vi "CalculateInputString_v2.vi"(1 "InputString":string="1 + 2 * 4") -> (0 "result":dbl format="%.2f")   [LabVIEW 2018]
uses:
  <vilib>/gmath/NI_Gmath.lvlib
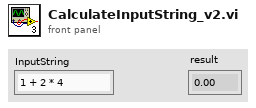
[diagram p1: front panel]
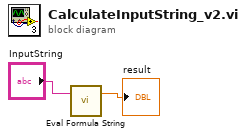
[diagram p0: block diagram]
diagram:
  n1 = call <vilib>:"Eval Formula String.vi"("formula"="InputString") -> ("y value"=→"result":dbl)  [unwired: 1 in, 1 out]
